vi "nirviGetTickCount.vi"() -> (0 "Tick Count(Ticks)":u32)   [LabVIEW 2017]
doc: "Returns the value of a free running counter in the units specified. The output and internal counter are both of the configured width."
panel:
  in  "Counter Units":u16(ring) items=["Ticks", "uSec", "mSec"]
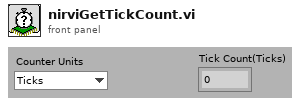
[diagram p1: front panel]
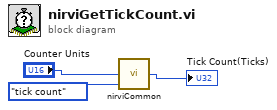
[diagram p0: block diagram]
diagram:
  n1 = call <vilib>:"nirviCommon.vi"("Action"=enum16{"wait", "wait multiple", "tick count"}."tick count", "Counter Units"="Counter Units") -> ("Tick Count(uSec)"=→"Tick Count(Ticks)":u32)  [unwired: 1 in]
